vi "Registry Simplify Data Type.vi"(4 "data type":T1(ring)) -> (1 "simple data type":enum16{"String", "Binary", "DWORD"}(ring))   [LabVIEW 2020]
doc: "Maps the Windows Registry data type to one of the following: String, Binary, or DWORD."
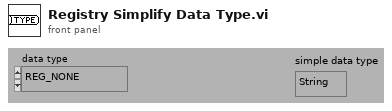
[diagram p1: front panel]
types:
  T1 = enum32{"REG_NONE", "REG_SZ", "REG_EXPAND_SZ", "REG_BINARY", "REG_DWORD_LITTLE_ENDIAN", "REG_DWORD_BIG_ENDIAN", "REG_LINK", "REG_MULTI_SZ", "REG_RESOURCE_LIST", "REG_FULL_RESOURCE_DESCRIPTOR", "REG_RESOURCE_REQUIREMENTS_LIST"}
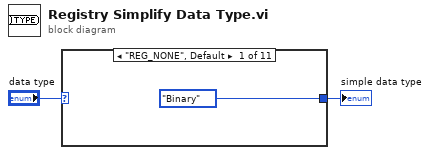
[diagram p0: block diagram]
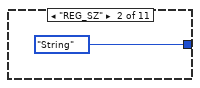
[diagram p2: hidden frame]
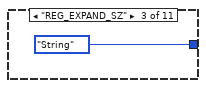
[diagram p3: hidden frame]
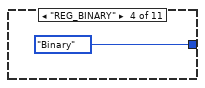
[diagram p4: hidden frame]
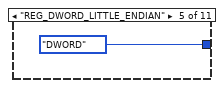
[diagram p5: hidden frame]
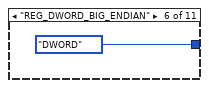
[diagram p6: hidden frame]
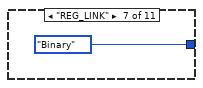
[diagram p7: hidden frame]
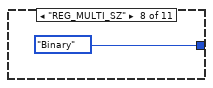
[diagram p8: hidden frame]
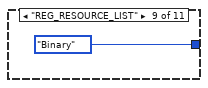
[diagram p9: hidden frame]
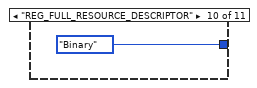
[diagram p10: hidden frame]
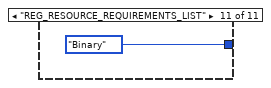
[diagram p11: hidden frame]
diagram:
  n1 = case shown="\"REG_NONE\", Default" "data type" {
    tunnel: [enum16{"String", "Binary", "DWORD"}."Binary" ("simplified data type") enum16{"String", "Binary", "DWORD"}."String" ("simplified data type") enum16{"String", "Binary", "DWORD"}."String" ("simplified data type") enum16{"String", "Binary", "DWORD"}."Binary" ("simplified data type") enum16{"String", "Binary", "DWORD"}."DWORD" ("simplified data type") enum16{"String", "Binary", "DWORD"}."DWORD" ("simplified data type") enum16{"String", "Binary", "DWORD"}."Binary" ("simplified data type") enum16{"String", "Binary", "DWORD"}."Binary" ("simplified data type") enum16{"String", "Binary", "DWORD"}."Binary" ("simplified data type") enum16{"String", "Binary", "DWORD"}."Binary" ("simplified data type") enum16{"String", "Binary", "DWORD"}."Binary" ("simplified data type")] -> w1
    frame "REG_NONE", Default {
    }
    frame "REG_SZ" {
    }
    frame "REG_EXPAND_SZ" {
    }
    frame "REG_BINARY" {
    }
    frame "REG_DWORD_LITTLE_ENDIAN" {
    }
    frame "REG_DWORD_BIG_ENDIAN" {
    }
    frame "REG_LINK" {
    }
    frame "REG_MULTI_SZ" {
    }
    frame "REG_RESOURCE_LIST" {
    }
    frame "REG_FULL_RESOURCE_DESCRIPTOR" {
    }
    frame "REG_RESOURCE_REQUIREMENTS_LIST" {
    }
  }
  "simple data type" <- w1
